vi "HandShaking.vi"(6 "Elapsed Time":u32, 8 "error in (no error)":errorcluster, 10 "Event Sources":T1, 11 "PreUUT in":refnum<class "PreUUT.lvclass">) -> (0 "error out":errorcluster, 3 "PreUUT out":refnum<class "PreUUT.lvclass">)   [LabVIEW 2021, in "OPC UA.lvlib" / "PreUUT.lvclass"]
uses:
  PreUUT.lvclass
  PreUUT.lvclass/PreUUT.ctl
  OPC UA/OPC UA.lvclass
  69382981-21da-416f-aaa9-716e16b0eed1.vi
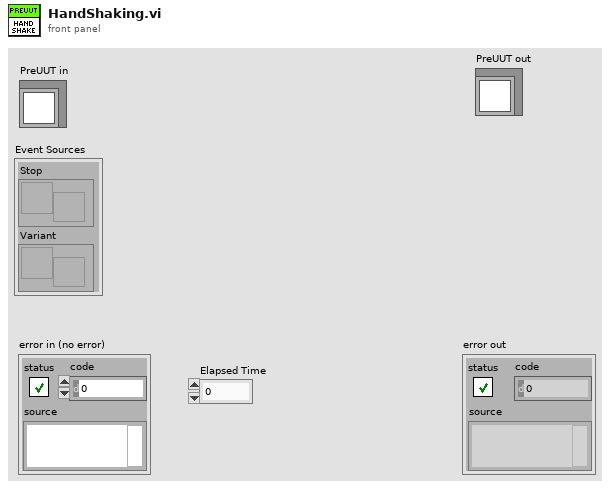
[diagram p1: front panel]
types:
  T1 = cluster{"Stop":refnum<user-event>, "Variant":refnum<user-event>}
  T2 = typedef "PreUUT.lvclass/Rx PreUUT.ctl" = cluster{"NestStatus":bool, "PalletID":u32, "Start":bool, "BarcodeData":string, "FaultCode":u32, "Stop":bool}
  T3 = typedef "OPC UA.lvlib/PreUUT.lvclass/Tx PreUUT.ctl" = cluster{"Online":bool, "Ready":bool, "Fault":bool, "Timeout":bool, "Results":u32, "StepNo":u32, "TestRunning":bool, "ResultsReady":bool, "Heartbeat":bool}
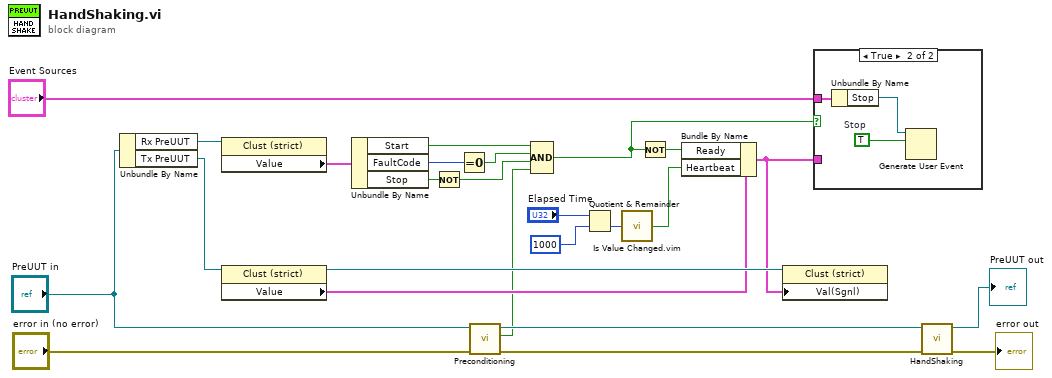
[diagram p0: block diagram]
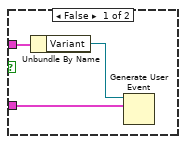
[diagram p2: hidden frame]
diagram:
  n1 = Unbundle By Name("PreUUT in") -> ("Rx PreUUT"=w23:refnum<vi>, "Tx PreUUT"=w13:refnum<vi>)
  n2 = property class="Clust (strict)"(reference=w23) -> ("Value"=w14:T2)  [unwired: 1 in, 2 out]
  n3 = property class="Clust (strict)"(reference=w13) -> (reference out=w24:refnum<vi>, "Value"=w22:T3)  [unwired: 1 in, 1 out]
  n4 = Unbundle By Name(w14) -> ("Start"=w15:bool, "FaultCode"=w17:u32, "Stop"=w18:bool)
  n5 = Not(x=w18) -> (.not. x?=w19:bool)
  n6 = Equal To 0?(x=w17) -> (x = 0?=w16:bool)
  n7 = call "Preconditioning.vi"("error in (no error)"="error in (no error)", "PreUUT in"="PreUUT in") -> ("error out"=w5:errorcluster, "Preconditioning"=w8:bool, "PreUUT out"=w9:refnum<class "PreUUT.lvclass">)  [unwired: 7 in]
  n8 = Compound Arithmetic op=AND(w15, w16, w19, w8) -> (w6:bool)
  n9 = Quotient & Remainder(x="Elapsed Time", y=u32 1000) -> (floor(x/y)=w4:u32)  [unwired: 1 out]
  n10 = call "Is Value Changed.vim"("value"=w4) -> ("changed or first call?"=w1:bool)
  n11 = Not(x=w6) -> (.not. x?=w21:bool)
  n12 = Bundle By Name(cluster=w22, "Ready"=w21, "Heartbeat"=w1) -> (w7:T3)
  n13 = property class="Clust (strict)"(reference=w24, "Val(Sgnl)"=w7) -> ()  [unwired: 1 in, 2 out]
  n14 = case shown="True" w6 {
    tunnel: w7 -> [w28 _]
    tunnel: "Event Sources" -> [w27 w31]
    frame False {
      n15 = Unbundle By Name(w27) -> ("Variant"=w26:refnum<user-event>)
      n16 = Generate User Event(user event=w26, event data cluster=w28) -> ()  [unwired: 2 in, 2 out]
    }
    frame True {
      w29 = TRUE  # Stop
      n17 = Unbundle By Name(w31) -> ("Stop"=w30:refnum<user-event>)
      n18 = Generate User Event(user event=w30, event data cluster=w29) -> ()  [unwired: 2 in, 2 out]
    }
  }
  n19 = call-parent "HandShaking.vi"("error in (no error)"=w5, "OPC UA in"=w9) -> ("error out"=→"error out":errorcluster, "OPC UA out"=→"PreUUT out":refnum<class "PreUUT.lvclass">)  [unwired: 8 in]
